vi "plot.volumes.vi"(4 "plot end":timestamp, 5 "Show Issues":bool, 6 "plot start":timestamp, 7 "picture in":picture, 9 "Width":u32, 10 "rows":T1(array[cluster]), 11 "volume objects":cluster{"Array":T2[]}[](array[cluster])) -> (1 "names":string[](array[string]), 2 "cells":T1(array[cluster]), 3 "picture":picture)   [LabVIEW 2024]
uses:
  CV_Shared_Library/volume.object--cluster.ctl
  CV_Shared_Library/volume.type--enum.ctl
  comic_manager/TypeDefs/issue.display--cluster.ctl
  CV_Shared_Library/CV_Shared_Library.lvlib
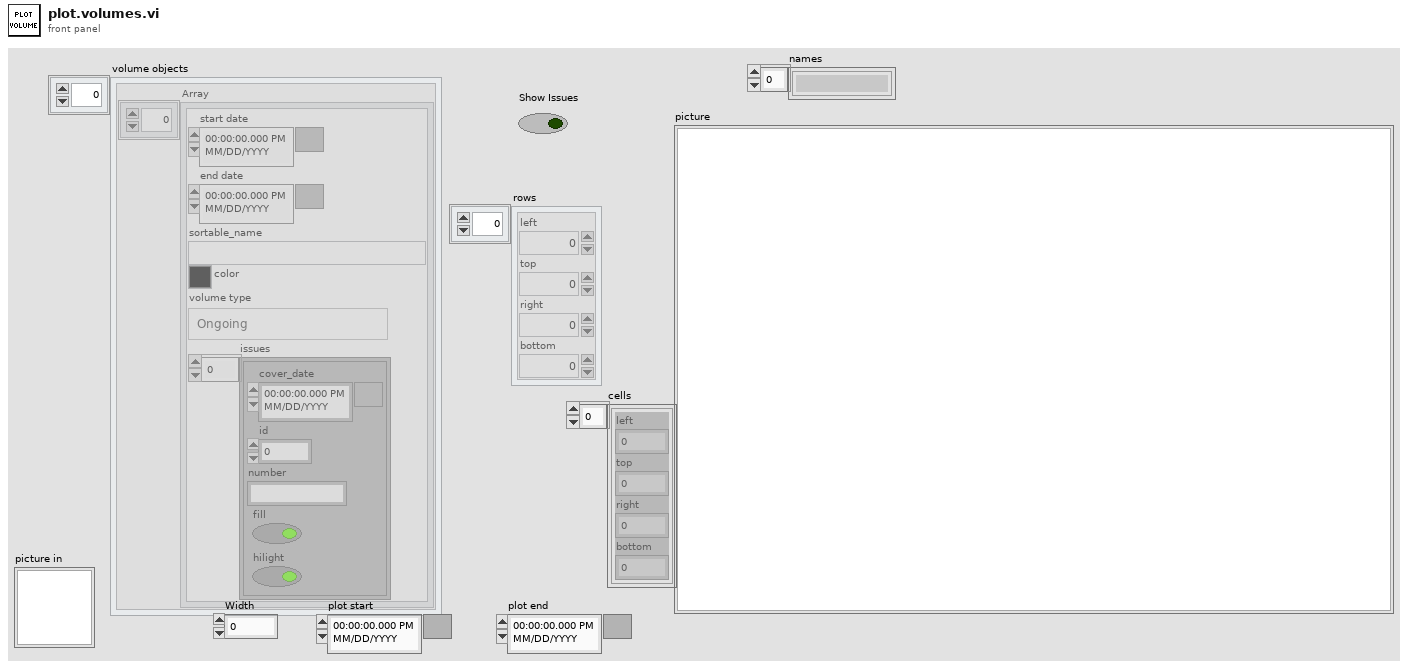
[diagram p1: front panel]
types:
  T1 = cluster{"left":i16, "top":i16, "right":i16, "bottom":i16}[]
  T2 = typedef "CV_Shared_Library.lvlib/volume.object--cluster.ctl" = cluster{"start date":timestamp, "end date":timestamp, "sortable_name":string, "color":u32, "volume type":T3, "issues":T4[]}
  T3 = typedef "CV_Shared_Library.lvlib/volume.type--enum.ctl" = enum16{"Ongoing", "Limited Series", "Annual", "One Shot", "Reprint/Document", "Star Comics", "Epic Comics"}
  T4 = typedef "CV_Shared_Library.lvlib/issue.display--cluster.ctl" = cluster{"cover_date":timestamp, "id":i32, "number":string, "fill":bool, "hilight":bool}
  T5 = cluster{"left":i16, "top":i16, "right":i16, "bottom":i16}
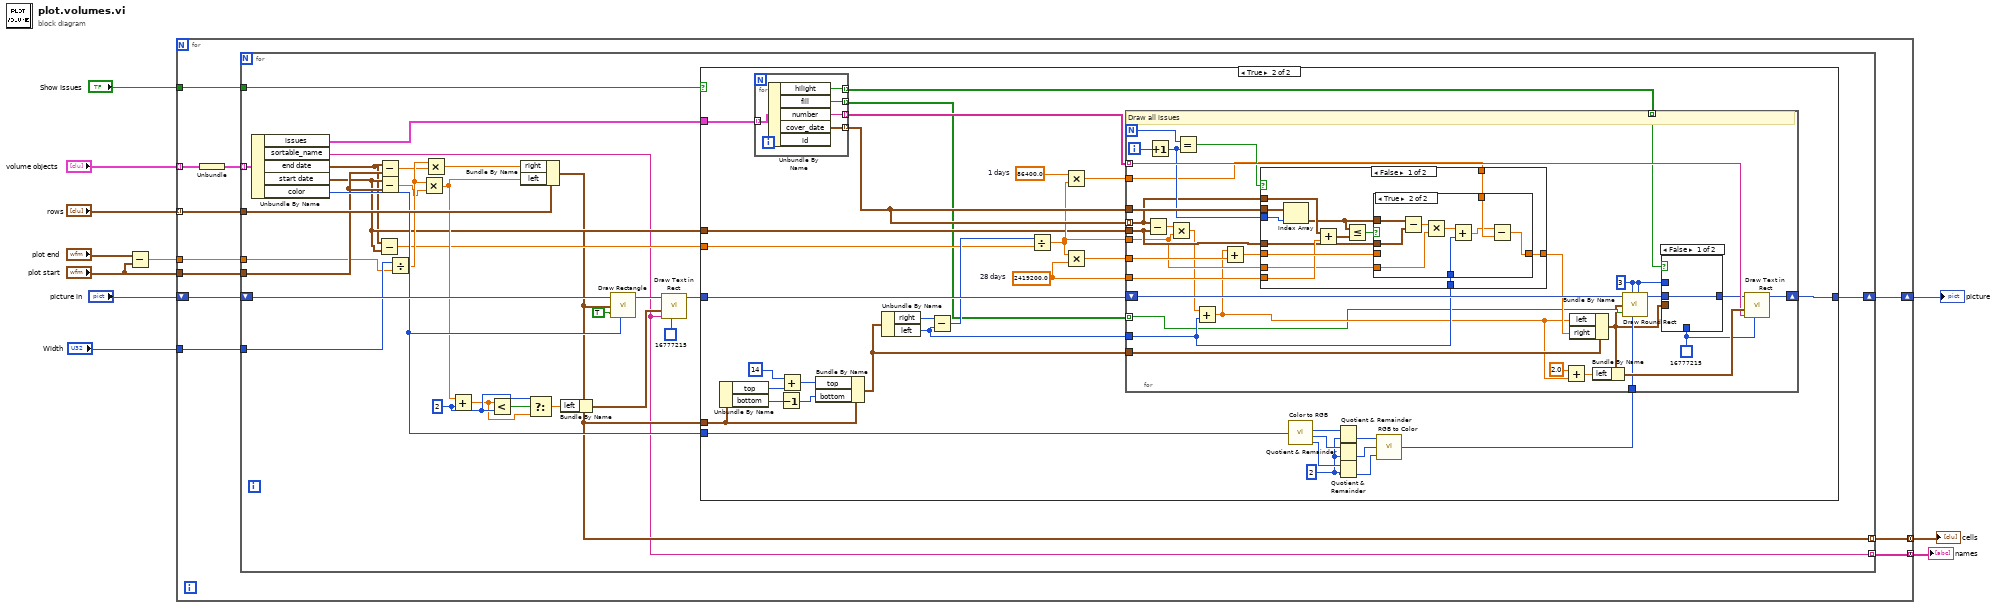
[diagram p0: block diagram]
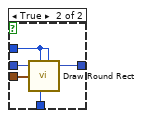
[diagram p3: hidden frame]
diagram:
  n1 = Subtract(x="plot end", y="plot start") -> (x-y=w4:dbl)
  n2 = for {
    tunnel: "volume objects" -> [w22] mode=indexing
    tunnel: "rows" -> [w20] mode=indexing
    tunnel: "plot start" -> [w19]
    tunnel: "Width" -> [w18]
    shift-right: [w16] -> w8
    shift-left: "picture in" -> [w17]
    tunnel: w4 -> [w15]
    tunnel: [w14] -> w3 mode=concatenating
    tunnel: [w13] -> w2 mode=concatenating
    tunnel: "Show Issues" -> [w12]
    n3 = Unbundle(w22) -> ("Array"=w21:T2[])
    n4 = for {
      tunnel: w21 -> [w51] mode=indexing
      tunnel: w20 -> [w49]
      tunnel: w19 -> [w31]
      tunnel: w18 -> [w36]
      shift-right: [w41] -> w16
      shift-left: w17 -> [w48]
      tunnel: w15 -> [w29]
      tunnel: [w25] -> w14 mode=indexing
      tunnel: [w24] -> w13 mode=indexing
      tunnel: w12 -> [w23]
      w39 = i16 2 ("left")
      n5 = Unbundle By Name(w51) -> ("issues"=w50:T4[], "sortable_name"=w24:string, "end date"=w27:timestamp, "start date"=w28:timestamp, "color"=w42:u32)
      n6 = Subtract(x=w27, y=w28) -> (x-y=w26:dbl)
      n7 = Subtract(x=w27, y=w31) -> (x-y=w34:dbl)
      n8 = Subtract(x=w28, y=w31) -> (x-y=w30:dbl)
      n9 = Divide(x=w36, y=w29) -> (x/y=w35:dbl)
      n10 = Multiply(x=w35, y=w30) -> (x*y=w32:dbl)
      n11 = Multiply(x=w35, y=w34) -> (x*y=w33:dbl)
      n12 = Add(x=w32, y=w39) -> (x+y=w38:dbl)
      n13 = Less?(x=w38, y=w39) -> (x < y?=w40:bool)
      n14 = Bundle By Name(cluster=w49, "right"=w33, "left"=w32) -> (w25:T5)
      n15 = Select(t=w39, s=w40, f=w38) -> (s? t:f=w37:dbl)
      n16 = Bundle By Name(cluster=w25, "left"=w37) -> (w45:T5)
      n17 = call <vilib>:"Draw Rectangle.vi"("picture"=w48, "rect"=w25, "fill?(F)"=TRUE, "color(black)"=w42) -> ("new picture"=w46:picture)  [unwired: 5 in]
      n18 = call <vilib>:"Draw Text in Rect.vi"("text color(black)"=u32 16777215, "text"=w24, "rect"=w45, "picture"=w46) -> ("new picture"=w43:picture)  [unwired: 7 in]
      n19 = case shown="True" w23 {
        tunnel: w50 -> [_ w85]
        tunnel: w43 -> [w52 w84]
        tunnel: w42 -> [_ w65]
        tunnel: [w52 w63] -> w41
        tunnel: w28 -> [_ w57]
        tunnel: w26 -> [_ w56]
        tunnel: w25 -> [_ w55]
        frame False {
        }
        frame True {
          w69 = u8 2 ("y")
          w73 = 2419200.0  # 28 days
          w76 = 86400.0  # 1 days
          n20 = Unbundle By Name(w55) -> ("top"=w82:i16, "bottom"=w80:i16)
          n21 = for {
            tunnel: w85 -> [w152] mode=indexing
            tunnel: [w151] -> w83 mode=indexing
            tunnel: [w150] -> w77 mode=indexing
            tunnel: [w149] -> w54 mode=indexing
            tunnel: [w148] -> w53 mode=indexing
            n22 = Unbundle By Name(w152) -> ("hilight"=w148:bool, "fill"=w149:bool, "number"=w151:string, "cover_date"=w150:timestamp)  [unwired: 1 out]
          }
          n23 = Decrement(x=w80) -> (x-1=w78:i16)
          n24 = Add(x=i16 14, y=w82) -> (x+y=w79:i16)
          n25 = Bundle By Name(cluster=w55, "top"=w79, "bottom"=w78) -> (w61:T5)
          n26 = Unbundle By Name(w61) -> ("right"=w60:i16, "left"=w59:i16)
          n27 = Subtract(x=w60, y=w59) -> (x-y=w58:i16)
          n28 = Divide(x=w58, y=w56) -> (x/y=w62:dbl)
          n29 = Multiply(x=w76, y=w62) -> (x*y=w75:dbl)
          n30 = Multiply(x=w62, y=w73) -> (x*y=w74:dbl)
          n31 = call <vilib>:"Color to RGB.vi"("Color"=w65) -> ("R"=w72:u8, "G"=w71:u8, "B"=w70:u8)  [unwired: 1 out]
          n32 = Quotient & Remainder(x=w72, y=w69) -> (floor(x/y)=w68:u8)  [unwired: 1 out]
          n33 = Quotient & Remainder(x=w71, y=w69) -> (floor(x/y)=w67:u8)  [unwired: 1 out]
          n34 = Quotient & Remainder(x=w70, y=w69) -> (floor(x/y)=w66:u8)  [unwired: 1 out]
          n35 = call <vilib>:"RGB to Color.vi"("B"=w66, "G"=w67, "R"=w68) -> ("Color"=w64:u32)
          n36 = for {
            N -> [w106]
            tunnel: w62 -> [w97]
            tunnel: w57 -> [w98]
            tunnel: w74 -> [w116]
            tunnel: w61 -> [w115]
            shift-right: [w111] -> w63
            shift-left: w84 -> [w114]
            tunnel: w83 -> [w109] mode=indexing
            tunnel: w77 -> [w99] mode=indexing
            tunnel: w64 -> [w108]
            tunnel: w77 -> [w102]
            tunnel: w75 -> [w96]
            tunnel: w73 -> [w100]
            tunnel: w59 -> [w94]
            tunnel: w54 -> [w92] mode=indexing
            tunnel: w53 -> [w91] mode=indexing
            i -> [w107]
            w89 = u32 16777215 ("text color(black)")
            w90 = i16 3 ("oval width")
            # "Draw all issues"
            n37 = Subtract(x=w99, y=w98) -> (x-y=w117:dbl)
            n38 = Increment(x=w107) -> (x+1=w101:i32)
            n39 = Multiply(x=w117, y=w97) -> (x*y=w95:dbl)
            n40 = Equal?(x=w106, y=w101) -> (x = y?=w105:bool)
            n41 = Add(x=w95, y=w94) -> (x+y=w93:dbl)
            n42 = Add(x=w93, y=w116) -> (x+y=w103:dbl)
            n43 = case shown="False" w105 {
              tunnel: [w133 w147] -> w104
              tunnel: w103 -> [w132 w147]
              tunnel: w102 -> [w136 _]
              tunnel: w101 -> [w135 _]
              tunnel: w100 -> [w131 _]
              tunnel: w99 -> [w129 _]
              tunnel: w98 -> [w127 _]
              tunnel: w97 -> [w126 _]
              tunnel: w96 -> [w125 _]
              tunnel: w94 -> [w124 _]
              frame False {
                n44 = Index Array(array=w136, index=w135) -> (element=w128:timestamp)
                n45 = Add(x=w129, y=w131) -> (x+y=w130:timestamp)
                n46 = Less Or Equal?(x=w128, y=w130) -> (x <= y?=w134:bool)
                n47 = case shown="True" w134 {
                  tunnel: [w137 w141] -> w133
                  tunnel: w132 -> [w137 _]
                  tunnel: w128 -> [_ w146]
                  tunnel: w127 -> [_ w145]
                  tunnel: w126 -> [_ w143]
                  tunnel: w125 -> [_ w142]
                  tunnel: w124 -> [_ w138]
                  frame False {
                  }
                  frame True {
                    n48 = Subtract(x=w146, y=w145) -> (x-y=w144:dbl)
                    n49 = Multiply(x=w144, y=w143) -> (x*y=w140:dbl)
                    n50 = Add(x=w140, y=w138) -> (x+y=w139:dbl)
                    n51 = Subtract(x=w139, y=w142) -> (x-y=w141:dbl)
                  }
                }
              }
              frame True {
              }
            }
            n52 = Add(x=2.0, y=w93) -> (x+y=w112:dbl)
            n53 = Bundle By Name(cluster=w115, "left"=w93, "right"=w104) -> (w88:T5)
            n54 = Bundle By Name(cluster=w88, "left"=w112) -> (w110:T5)
            n55 = call <vilib>:"Draw Round Rect.vi"("picture"=w114, "oval width"=w90, "rect"=w88, "fill?(F)"=w92, "color(black)"=w108, "oval height"=w90) -> ("new picture"=w87:picture)  [unwired: 3 in]
            n56 = case shown="False" w91 {
              tunnel: w90 -> [_ w123]
              tunnel: w89 -> [_ w122]
              tunnel: w88 -> [_ w121]
              tunnel: w87 -> [w118 w120]
              tunnel: [w118 w119] -> w86
              frame False {
              }
              frame True {
                n57 = call <vilib>:"Draw Round Rect.vi"("picture"=w120, "oval width"=w123, "rect"=w121, "color(black)"=w122, "oval height"=w123) -> ("new picture"=w119:picture)  [unwired: 4 in]
              }
            }
            n58 = call <vilib>:"Draw Text in Rect.vi"("text color(black)"=w89, "text"=w109, "rect"=w110, "picture"=w86) -> ("new picture"=w111:picture)  [unwired: 7 in]
          }
        }
      }
    }
  }
  "picture" <- w8
  "cells" <- w3
  "names" <- w2
